vi "Set Serializer.vi"(8 "error in (no error)":errorcluster, 10 "Serializer (default: Flattened String)":refnum<class "Serializer.lvclass">, 11 "MQTT_Base":refnum<class "MQTT_Base.lvclass">) -> (0 "error out":errorcluster, 3 "MQTT_Base out":refnum<class "MQTT_Base.lvclass">)   [LabVIEW 2013, in "MQTT Base.lvlib" / "MQTT_Base.lvclass"]
uses:
  MQTT_Base.lvclass
  <vilib>/LabVIEW Open Source Project/OpenSerializer/Serializer/Serializer.lvclass
  <vilib>/LabVIEW Open Source Project/OpenSerializer/Serializer.FlattenedString/Serializer.FlattenedString.lvclass
  MQTT_Base.lvclass/MQTT_Base.ctl
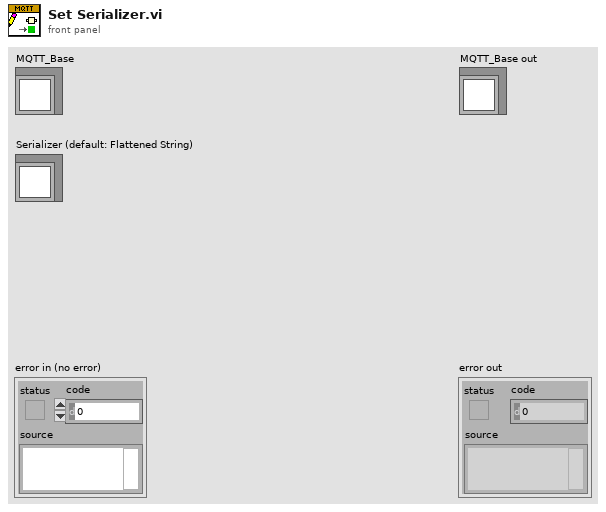
[diagram p1: front panel]
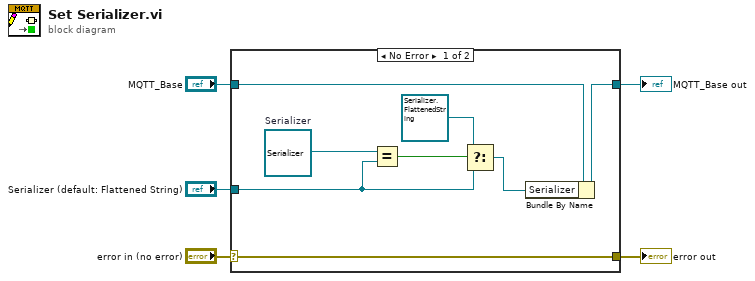
[diagram p0: block diagram]
diagram:
  n1 = case shown="No Error" "error in (no error)" {
    selector: "error in (no error)" -> [w13 w14]
    tunnel: [w13 w14] -> w4
    tunnel: [w8 w15] -> w2
    tunnel: "MQTT_Base" -> [w12 w15]
    tunnel: "Serializer (default: Flattened String)" -> [w10 _]
    frame No Error {
      w7 = refnum<class "Serializer.lvclass"> refnum  # Serializer
      n2 = Equal?(x=w7, y=w10) -> (x = y?=w11:bool)
      n3 = Select(t=refnum<class "Serializer.FlattenedString.lvclass"> refnum ("FlattenedString Serializer"), s=w11, f=w10) -> (s? t:f=w9:refnum<class "Serializer.lvclass">)
      n4 = Bundle By Name(cluster=w12, "Serializer"=w9) -> (w8:refnum<class "MQTT_Base.lvclass">)
    }
    frame Error {
    }
  }
  "error out" <- w4
  "MQTT_Base out" <- w2
